vi "Day7-2.vi"() -> ()   [LabVIEW 2021]
uses:
  4c816eb8-5152-4e16-8102-76167b0c092a.vi
  <vilib>/Comparison/Less/Less Functor/Less Functor.lvclass
panel:
  out "Array 2":cluster{"path":path, i32}[](array[cluster])
  out "x-y":i32
  out "sorted array":cluster{i32, "path":path}[](array[cluster])
  out "sum 2":i32
  out "Array":cluster{"path":path, i32}[](array[cluster])
  out "array":string[][](array[string])
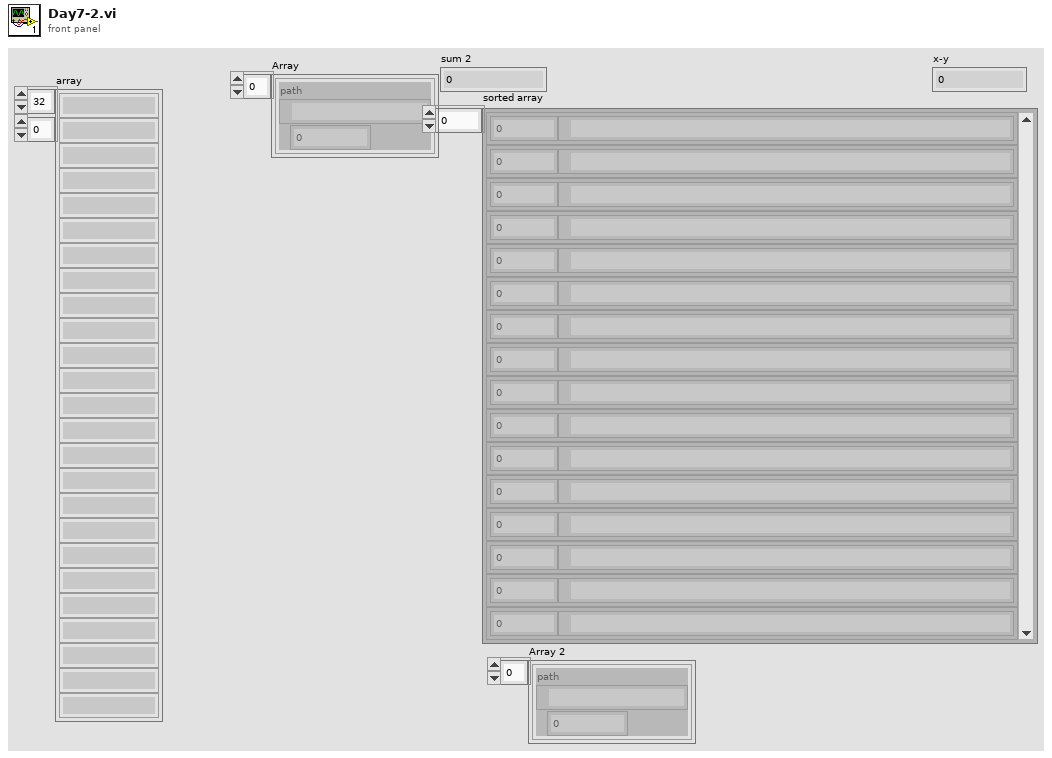
[diagram p1: front panel]
types:
  T1 = map{path, cluster{"parent directory":string, "subdirectories":string[], "contained files":cluster{"file name":string, "file size":i32}[]}}
  T2 = cluster{"parent direcotry":string, "subdirectories":string[], "contained files":cluster{"file name":string, "file size":i32}[]}
  T3 = cluster{"trimmed string":string, "file size":i32}[]
  T4 = cluster{"parent directory":string, "subdirectories":string[], "contained files":cluster{"file name":string, "file size":i32}[]}
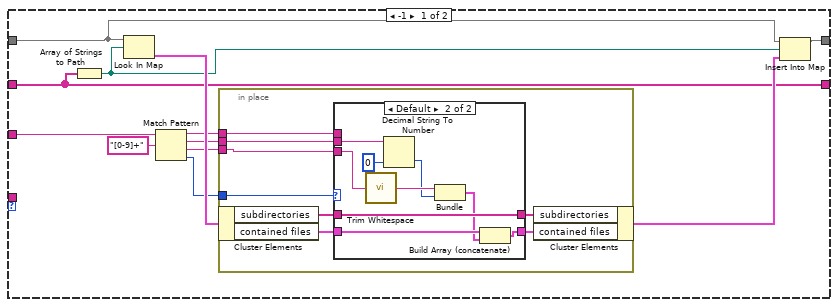
[diagram p2: hidden frame]
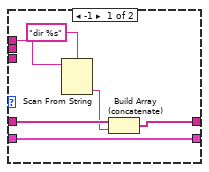
[diagram p3: hidden frame]
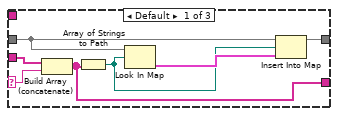
[diagram p5: hidden frame]
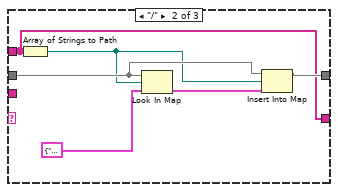
[diagram p6: hidden frame]
diagram:
  w14 = T1 {}  # Size: 0
  (unwired) "- / (dir)\n  - a (dir)\n    - e (dir)\n      - i (file, size=584)\n    - f (file, size=29116)\n    - g (file, size=2557)\n    - h.lst (file, size=62596)\n  - b.txt (file, size=14848514)\n  - c.dat (file, size=8504156)\n  - d (dir)\n    - j (file, size=4060174)\n    - d.log (file, size=8033020)\n    - d.ext (file, size=5626152)\n    - k (file, size=7214296)"
  # "directory properties\n - parent directory\n - subdirectories\n - contained files"
  # "active directory"
  n1 = Spreadsheet String To Array(format string="%s" ("spreadsheet string"), spreadsheet string="$ cd /\n$ ls\ndir ccjp\n328708 hglnvs.bsh\ndir hpsnpc\ndir pcb\ndir pntzm\ndir pzg\ndir thfgwwsp\n$ cd ccjp\n$ ls\n159990 dlz\ndir mbtsvblj\n165076 nppbjl.qhg\n$ cd mbtsvblj\n$ ls\n34806 frqsf.nsv\ndir ppq\ndir ptht\ndir rgmvdwt\n$ cd ppq\n$ ls\n266252 dhzp\n$ cd ..\n$ cd ptht\n$ ls\ndir jbnj\ndir zcbnwhzd\n$ cd jbnj\n$ ls\ndir clscr\n145780 zwtwf.zfz\n$ cd clscr\n$ ls\n249531 dhzp\n$ cd ..\n$ cd ..\n$ cd zcbnwhzd\n$ ls\ndir mbtsvblj\n$ cd mbtsvblj\n$ ls\n258527 pjhvzjt.brz\n$ cd ..\n$ cd ..\n$ cd ..\n$ cd rgmvdwt\n$ ls\n166021 hdb\n115350 ljpzpdbf\n$ cd ..\n$ cd ..\n$ cd ..\n$ cd hpsnpc\n$ ls\n6334 bfdfbrh.vff\n311949 qphlw.whm\n$ cd ..\n$ cd pcb\n$ ls\ndir ccjp\n201615 gbpzf.gmg\ndir lhth\n319302 lrmj.rmm\ndir mwl\n303062 pvftq\n$ cd ccjp\n$ ls\n10932 ccjp\n80040 jjcggmr.ljs\n299982 jrqwhsn.ptv\n280655 ljpzpdbf\n268430 mdvvj.dlf\ndir mvhhlg\ndir ppfq\ndir rdgngdm\ndir smftmb\ndir tqwchhd\n$ cd mvhhlg\n$ ls\n146902 fwhcbfr.shd\n$ cd ..\n$ cd ppfq\n$ ls\n263452 hdb\n$ cd ..\n$ cd rdgngdm\n$ ls\n46355 wlgshdgl\n$ cd ..\n$ cd smftmb\n$ ls\n56834 mhs\n325038 ppmtvcj\ndir rzcmwl\n194645 ztwqq.jfw\n$ cd rzcmwl\n$ ls\ndir btfhswwf\ndir jrd\ndir ndzfvl\n$ cd btfhswwf\n$ ls\n62811 ccjp.clj\n$ cd ..\n$ cd jrd\n$ ls\n184948 fqqg.pfc\ndir mshf\n136894 nbvbr\n$ cd mshf\n$ ls\n314602 ppmtvcj\n$ cd ..\n$ cd ..\n$ cd ndzfvl\n$ ls\n43177 hhcfpnmg.njm\n$ cd ..\n$ cd ..\n$ cd ..\n$ cd tqwchhd\n$ ls\n294014 dlz\n122061 ljpzpdbf\n54178 ppmtvcj.wlp\ndir trm\ndir zcbnwhzd\n$ cd trm\n$ ls\n279737 ccjp.mhz\n$ cd ..\n$ cd zcbnwhzd\n$ ls\n88477 dhnwjlzj\n143989 dhzp\n$ cd ..\n$ cd ..\n$ cd ..\n$ cd lhth\n$ ls\n79532 tlls\n$ cd ..\n$ cd mwl\n$ ls\ndir frc\ndir lqqqppm\n178576 prpjmrw\n$ cd frc\n$ ls\ndir cvm\n244013 dhzp\n29325 gnh\n264555 hdb\n$ cd cvm\n$ ls\n196619 hhcfpnmg.njm\n$ cd ..\n$ cd ..\n$ cd lqqqppm\n$ ls\ndir jdznl\n38505 nqv\n$ cd jdznl\n$ ls\n85492 ctt\n228912 dfbgtqj.vsb\n136077 nnwgd.vjn\n254459 zrrzsfss\n$ cd ..\n$ cd ..\n$ cd ..\n$ cd ..\n$ cd pntzm\n$ ls\ndir hnnhdd\ndir mbtsvblj\ndir vmdlwdj\n$ cd hnnhdd\n$ ls\n35908 fjp\n119221 ljpzpdbf\n210488 whhpztz.lgt\n$ cd ..\n$ cd mbtsvblj\n$ ls\ndir clfpc\ndir csqcnmtc\n18524 mbtsvblj\ndir zcrrtlh\n$ cd clfpc\n$ ls\ndir jffq\ndir qpsfrhld\n89569 tdzfqpz.wvs\n$ cd jffq\n$ ls\ndir dpngpgr\ndir htbf\n$ cd dpngpgr\n$ ls\n128899 ccjp.nbs\n$ cd ..\n$ cd htbf\n$ ls\n90381 ljpzpdbf\n$ cd ..\n$ cd ..\n$ cd qpsfrhld\n$ ls\ndir bgrb\ndir ddtlcfz\n54115 dlz\n154299 hhcfpnmg.njm\n59452 jwc.pwg\ndir mbtsvblj\n$ cd bgrb\n$ ls\n119046 ccjp.zmf\ndir qsnng\n$ cd qsnng\n$ ls\n195412 vjdh.cqv\n$ cd ..\n$ cd ..\n$ cd ddtlcfz\n$ ls\ndir ftfch\n26717 mbtsvblj\n157679 mbtsvblj.rfb\n299928 qmg\ndir trq\ndir wjhjlpr\n$ cd ftfch\n$ ls\n50242 dhzp\n58846 dlz\ndir hhwsrzhv\n$ cd hhwsrzhv\n$ ls\ndir bjnn\n67610 dhzp\ndir mbtsvblj\n205664 tmcfmshb\n$ cd bjnn\n$ ls\n199806 dlz\n$ cd ..\n$ cd mbtsvblj\n$ ls\ndir ffzjcshp\n$ cd ffzjcshp\n$ ls\ndir ppmtvcj\n$ cd ppmtvcj\n$ ls\n184744 dlz\n$ cd ..\n$ cd ..\n$ cd ..\n$ cd ..\n$ cd ..\n$ cd trq\n$ ls\n278471 ccjp\n$ cd ..\n$ cd wjhjlpr\n$ ls\ndir wzwqrfhv\n$ cd wzwqrfhv\n$ ls\n262877 ccjp\n$ cd ..\n$ cd ..\n$ cd ..\n$ cd mbtsvblj\n$ ls\n243142 ccjp.szb\n306673 lmstdpfc.nww\ndir nlsprnh\ndir nmzwtwwc\ndir rbpbl\n$ cd nlsprnh\n$ ls\n200708 stbjphg.hcs\n$ cd ..\n$ cd nmzwtwwc\n$ ls\n323366 vzq.pcj\n$ cd ..\n$ cd rbpbl\n$ ls\n59872 fmnmsjr.svf\n$ cd ..\n$ cd ..\n$ cd ..\n$ cd ..\n$ cd csqcnmtc\n$ ls\n16652 ccjp\ndir fsfd\n37144 hdb\ndir mbtsvblj\ndir mwl\n66387 nljlpbjq\ndir ppmtvcj\n120839 rgclgwnq\n$ cd fsfd\n$ ls\n105721 qqvchq.mwh\n$ cd ..\n$ cd mbtsvblj\n$ ls\ndir cdzgtll\ndir dfgd\ndir fbfr\n165975 mbtsvblj\n174541 ppmtvcj\ndir vwgrpswj\n$ cd cdzgtll\n$ ls\n163523 dhzp\n124219 dlz\n199796 hdb\n$ cd ..\n$ cd dfgd\n$ ls\n173064 ccjp.cbt\ndir cdqc\ndir fzrm\ndir grcs\n87000 mbtsvblj.zrl\ndir njvgs\ndir ppmtvcj\n210984 rhtslcwt.wgt\ndir vws\n$ cd cdqc\n$ ls\n178924 hdb\n$ cd ..\n$ cd fzrm\n$ ls\ndir bjwtbc\n211229 dhzp\ndir dtslj\n76461 mbtsvblj.mtw\n317618 mmz.mqq\ndir mwl\n163587 vwgq\n$ cd bjwtbc\n$ ls\n9891 hhcfpnmg.njm\ndir mwl\n$ cd mwl\n$ ls\n203337 glwp.dls\n112753 mwl.qph\n$ cd ..\n$ cd ..\n$ cd dtslj\n$ ls\n277817 hhcfpnmg.njm\n$ cd ..\n$ cd mwl\n$ ls\n90781 mhnrwpmg.svv\n$ cd ..\n$ cd ..\n$ cd grcs\n$ ls\n286144 rnfqhs\n$ cd ..\n$ cd njvgs\n$ ls\ndir bmhdth\ndir ccjp\ndir mwl\n$ cd bmhdth\n$ ls\n154455 ppmtvcj.hwq\n$ cd ..\n$ cd ccjp\n$ ls\n215864 fcwjtzhs.vqn\n$ cd ..\n$ cd mwl\n$ ls\n139000 fnjztz\n$ cd ..\n$ cd ..\n$ cd ppmtvcj\n$ ls\n45041 jzfnmdw.jms\ndir zstzfs\n$ cd zstzfs\n$ ls\ndir qsfsj\n$ cd qsfsj\n$ ls\n34771 rsv\n$ cd ..\n$ cd ..\n$ cd ..\n$ cd vws\n$ ls\n98036 pjs\n103603 szszjfv\n211083 ztd\n$ cd ..\n$ cd ..\n$ cd fbfr\n$ ls\ndir dshrpf\n216109 hbw.jhj\n319355 hdhl\ndir ltf\n210950 qstlgvb\ndir thhncv\n316300 zfgh\n$ cd dshrpf\n$ ls\ndir nll\ndir qrsg\n$ cd nll\n$ ls\n45935 flmvswv.rll\n4161 hhcfpnmg.njm\n82301 sww.dwj\ndir tqdmtp\n46608 tzrn.qrt\n101463 zcbnwhzd.mpm\n$ cd tqdmtp\n$ ls\n280430 dhzp\n$ cd ..\n$ cd ..\n$ cd qrsg\n$ ls\ndir htrvnvz\n$ cd htrvnvz\n$ ls\ndir mbtsvblj\n$ cd mbtsvblj\n$ ls\n235270 dlz\n$ cd ..\n$ cd ..\n$ cd ..\n$ cd ..\n$ cd ltf\n$ ls\ndir pcbc\ndir wwjnwbjj\ndir zcbnwhzd\n$ cd pcbc\n$ ls\n140010 mbtsvblj.hqd\n$ cd ..\n$ cd wwjnwbjj\n$ ls\ndir mwl\n$ cd mwl\n$ ls\ndir pddbdp\n$ cd pddbdp\n$ ls\n27497 dlz\n$ cd ..\n$ cd ..\n$ cd ..\n$ cd zcbnwhzd\n$ ls\n302364 nrgpwm.cbb\n$ cd ..\n$ cd ..\n$ cd thhncv\n$ ls\n299769 hdb\n$ cd ..\n$ cd ..\n$ cd vwgrpswj\n$ ls\ndir jgt\ndir mwl\n293673 mwl.pwl\n$ cd jgt\n$ ls\n282773 hhcfpnmg.njm\n$ cd ..\n$ cd mwl\n$ ls\n288944 jfnjdtr.ssj\n186368 wfr\ndir zrtvvf\n$ cd zrtvvf\n$ ls\n82162 gtz.gsc\n$ cd ..\n$ cd ..\n$ cd ..\n$ cd ..\n$ cd mwl\n$ ls\n98218 htc.qjr\ndir mghhqrtn\ndir qct\n$ cd mghhqrtn\n$ ls\n220446 dlz\n36230 pwwlwv.crn\n$ cd ..\n$ cd qct\n$ ls\n33534 hdb\n27140 jpwqvbs.mvr\n60637 mlqtp\n12143 nlvtp.qjn\n152733 nqjqzt\n$ cd ..\n$ cd ..\n$ cd ppmtvcj\n$ ls\ndir ccjp\n297245 zcbnwhzd\n$ cd ccjp\n$ ls\n128473 wcw.dng\n$ cd ..\n$ cd ..\n$ cd ..\n$ cd zcrrtlh\n$ ls\n27488 bcbnmhq\ndir dhsmmlt\ndir fgqbpcn\n$ cd dhsmmlt\n$ ls\n42514 cvfwqnfl\n252570 dlz\n145814 ppmtvcj.snb\n294613 rslsh.slv\n186477 vwd.spz\ndir wffbp\n$ cd wffbp\n$ ls\ndir mbtsvblj\ndir nvq\n150447 ppmtvcj.hzc\n34904 whzpsbqp.clq\ndir zcbnwhzd\n$ cd mbtsvblj\n$ ls\n65132 cmmlw.bmq\n310866 cqrtmpdp.pjq\ndir mbtsvblj\n212527 mbtsvblj.spw\n232198 ngmltt.qwl\ndir pbqh\ndir ppwgsp\ndir qqfsb\n223322 tzsmvh\n$ cd mbtsvblj\n$ ls\ndir bzpdz\ndir mbtsvblj\ndir pwnn\ndir zcbnwhzd\n$ cd bzpdz\n$ ls\n272769 gtmftv\n280597 hhcfpnmg.njm\n151008 nmgvrhr.mvp\n$ cd ..\n$ cd mbtsvblj\n$ ls\n64862 czn\n309781 dhzp\n253325 dlz\ndir dqnr\ndir fgd\n139779 ghtzv\n255567 rml.rhm\ndir srfzjfw\n$ cd dqnr\n$ ls\n302986 cjnwm.lrb\n158871 frhjlp.rnn\n180385 nrlmq\n$ cd ..\n$ cd fgd\n$ ls\n158213 msjrcl.dsh\n$ cd ..\n$ cd srfzjfw\n$ ls\ndir jfnd\n210830 ljpzpdbf\ndir mbtsvblj\ndir zcrrvpg\n$ cd jfnd\n$ ls\n300883 zvtdj.srv\n$ cd ..\n$ cd mbtsvblj\n$ ls\n287467 cjdm.whc\n233084 hpfgtnts\ndir zcbnwhzd\n$ cd zcbnwhzd\n$ ls\n79744 dlz\n$ cd ..\n$ cd ..\n$ cd zcrrvpg\n$ ls\ndir jrbcqlct\ndir srpm\n$ cd jrbcqlct\n$ ls\n325945 dlz\n$ cd ..\n$ cd srpm\n$ ls\n90698 ngw.fhm\n$ cd ..\n$ cd ..\n$ cd ..\n$ cd ..\n$ cd pwnn\n$ ls\n104826 ppmtvcj.jtm\n$ cd ..\n$ cd zcbnwhzd\n$ ls\n145508 fnr.dgt\n256683 gwdl.vfl\ndir mdv\n44255 mqdv.cdb\n79723 rgvcf\ndir sjdh\n88945 wdgq.hfm\ndir zpm\n$ cd mdv\n$ ls\n231290 dlz\n3468 hdb\n95091 mcm\n67779 mwl.ncb\ndir ppf\ndir rfwwtjdn\n143730 slrv.qdl\ndir sqbdvppf\n$ cd ppf\n$ ls\n73809 rgdtlp\n$ cd ..\n$ cd rfwwtjdn\n$ ls\n255306 dhzp\n306865 zbnmtcgr.ddf\n237019 zcbnwhzd.szn\n$ cd ..\n$ cd sqbdvppf\n$ ls\ndir ccjp\ndir mbtsvblj\n142955 str\ndir whtrbcqn\n93407 zcbnwhzd.ctr\n$ cd ccjp\n$ ls\n29914 cwtvtcnp.tft\n295537 rvlb\n$ cd ..\n$ cd mbtsvblj\n$ ls\n262652 ccjp.wbn\n297839 mbtsvblj.gnz\n249019 pqsqjg.vwr\n$ cd ..\n$ cd whtrbcqn\n$ ls\ndir ccjp\ndir hslmvvb\n51040 vzcsfcwf\n$ cd ccjp\n$ ls\n39489 slps\n$ cd ..\n$ cd hslmvvb\n$ ls\n148628 gpwnf.qtd\ndir jrl\n11814 qtjtsvgg.ltz\n$ cd jrl\n$ ls\ndir scwlmjzm\n$ cd scwlmjzm\n$ ls\n119717 vhpsrbzw.jnh\n$ cd ..\n$ cd ..\n$ cd ..\n$ cd ..\n$ cd ..\n$ cd ..\n$ cd sjdh\n$ ls\n43495 srwzspsl\n$ cd ..\n$ cd zpm\n$ ls\n137218 mwl.pzt\n$ cd ..\n$ cd ..\n$ cd ..\n$ cd pbqh\n$ ls\n202610 dlz\ndir vdrqc\n$ cd vdrqc\n$ ls\n202958 mzzmjrt\n$ cd ..\n$ cd ..\n$ cd ppwgsp\n$ ls\n248541 pzvtdl.lcc\n$ cd ..\n$ cd qqfsb\n$ ls\n211390 mbtsvblj.fvh\n241455 mwl.bzl\n$ cd ..\n$ cd ..\n$ cd nvq\n$ ls\n74730 hhcfpnmg.njm\n257109 ljpzpdbf\n8864 zcbnwhzd.ctj\n$ cd ..\n$ cd zcbnwhzd\n$ ls\n307501 ccjp\ndir dfgbztqr\ndir mwl\n248526 pmhtz\ndir rwmzdt\n$ cd dfgbztqr\n$ ls\n18261 hdb\ndir mwl\ndir ppmtvcj\n$ cd mwl\n$ ls\n36787 hdv.vfs\n283104 zrvbsht.fmm\n$ cd ..\n$ cd ppmtvcj\n$ ls\n208809 ljpzpdbf\n$ cd ..\n$ cd ..\n$ cd mwl\n$ ls\n195369 mgfvgw\n146522 mwl\n78589 sfthn\n$ cd ..\n$ cd rwmzdt\n$ ls\n10176 hdb\n$ cd ..\n$ cd ..\n$ cd ..\n$ cd ..\n$ cd fgqbpcn\n$ ls\n169227 dhzp\ndir dwsgcrz\n140391 pjjln.ngc\n162589 ppmtvcj.ngb\n199626 rcgbjn.wfv\ndir snrl\ndir vfnrs\n$ cd dwsgcrz\n$ ls\n300751 fjlw.wtp\n$ cd ..\n$ cd snrl\n$ ls\n16142 ccjp.jpw\n150389 cmbnljt.ljq\n52600 gqggd.dwm\n$ cd ..\n$ cd vfnrs\n$ ls\n217267 bwlpdfv.hzh\n$ cd ..\n$ cd ..\n$ cd ..\n$ cd ..\n$ cd vmdlwdj\n$ ls\n29199 bcgjdpj.qcj\n172894 jjgrcd.cvf\ndir ngpnmbqz\n296193 ppmtvcj.bfr\ndir tfvhhpn\n36476 wqzst.wcj\n$ cd ngpnmbqz\n$ ls\ndir gnsm\ndir ntsgrm\n$ cd gnsm\n$ ls\ndir rjzngs\ndir tvv\n$ cd rjzngs\n$ ls\ndir dpfcw\ndir spmhrb\n$ cd dpfcw\n$ ls\n181566 mgdjjd.pqg\n$ cd ..\n$ cd spmhrb\n$ ls\n163198 hhcfpnmg.njm\n$ cd ..\n$ cd ..\n$ cd tvv\n$ ls\n131443 hhcfpnmg.njm\n$ cd ..\n$ cd ..\n$ cd ntsgrm\n$ ls\n246786 dlz\n12841 pzbgrn\n$ cd ..\n$ cd ..\n$ cd tfvhhpn\n$ ls\n196923 dhzp\n$ cd ..\n$ cd ..\n$ cd ..\n$ cd pzg\n$ ls\n262706 ppbqssj.hjj\n$ cd ..\n$ cd thfgwwsp\n$ ls\ndir dsvc\ndir fbg\ndir flgmdj\n516 gwppndsl\ndir mwl\ndir qfhsr\ndir tgj\ndir wdmzc\n272804 zcbnwhzd\ndir zrfmzrl\n$ cd dsvc\n$ ls\n22089 dlz\n$ cd ..\n$ cd fbg\n$ ls\n289639 hhcfpnmg.njm\n$ cd ..\n$ cd flgmdj\n$ ls\n293793 fqrpf\n$ cd ..\n$ cd mwl\n$ ls\n159673 dhzp\ndir ftthgr\n270973 hhcfpnmg.njm\ndir jjrq\n279365 ljpzpdbf\ndir mglzfcq\n101769 pnz\n18964 rdl.wqf\n$ cd ftthgr\n$ ls\ndir ccrvnht\n170369 ljltl.slv\ndir mwl\ndir zqts\n65217 zvnhmqpz.cqb\n$ cd ccrvnht\n$ ls\n164437 hdb\n$ cd ..\n$ cd mwl\n$ ls\ndir cjsc\ndir zcbnwhzd\ndir zwzb\n$ cd cjsc\n$ ls\n91883 hhcfpnmg.njm\n203008 nfmvr\n$ cd ..\n$ cd zcbnwhzd\n$ ls\ndir mbtsvblj\n$ cd mbtsvblj\n$ ls\n187513 ljpzpdbf\n$ cd ..\n$ cd ..\n$ cd zwzb\n$ ls\n138631 ljpzpdbf\ndir sjngjp\n$ cd sjngjp\n$ ls\n52116 ccjp.ttc\n157900 fptzbpp.sdm\n89462 hhcfpnmg.njm\n$ cd ..\n$ cd ..\n$ cd ..\n$ cd zqts\n$ ls\n162402 hdb\n$ cd ..\n$ cd ..\n$ cd jjrq\n$ ls\ndir bffvw\ndir czbwf\n13447 dlz\ndir gjh\ndir hjs\n$ cd bffvw\n$ ls\n139679 dqqtq.lnb\ndir mwl\n13310 sjln.zgv\n243329 srmghrt.ffl\n72108 ssm.tph\n$ cd mwl\n$ ls\ndir fdlmfjt\ndir jms\n122108 nqwrj\n$ cd fdlmfjt\n$ ls\n75969 hdtbcsfc.vmz\n$ cd ..\n$ cd jms\n$ ls\n297556 hhcfpnmg.njm\n$ cd ..\n$ cd ..\n$ cd ..\n$ cd czbwf\n$ ls\n320541 ccjp\n$ cd ..\n$ cd gjh\n$ ls\n164281 dhzp\n286094 vjs\n$ cd ..\n$ cd hjs\n$ ls\ndir cbdzvd\n41353 ccjp\ndir gbs\n114686 hdb\ndir hmtpm\n278709 ljpzpdbf\ndir ppmtvcj\n292308 zcmlbbbc.mpp\n86096 zttwct\n$ cd cbdzvd\n$ ls\n153733 dhzp\n$ cd ..\n$ cd gbs\n$ ls\ndir nfnb\n$ cd nfnb\n$ ls\ndir hgm\n$ cd hgm\n$ ls\n233469 ljpzpdbf\n$ cd ..\n$ cd ..\n$ cd ..\n$ cd hmtpm\n$ ls\n14247 mwl\n$ cd ..\n$ cd ppmtvcj\n$ ls\ndir jcwhvcf\n241390 mwl\n$ cd jcwhvcf\n$ ls\n198254 wddq.rgp\n$ cd ..\n$ cd ..\n$ cd ..\n$ cd ..\n$ cd mglzfcq\n$ ls\ndir bsplglmj\n21700 fhflt.vgq\n56724 lpmcbzrj\n222733 qnbr\n256952 thvbqb.gtv\n$ cd bsplglmj\n$ ls\ndir zcbnwhzd\n$ cd zcbnwhzd\n$ ls\ndir mqzqz\n$ cd mqzqz\n$ ls\n75000 ppmtvcj\n$ cd ..\n$ cd ..\n$ cd ..\n$ cd ..\n$ cd ..\n$ cd qfhsr\n$ ls\n249770 gfv.cnw\n70204 qlvwhff.jhm\n$ cd ..\n$ cd tgj\n$ ls\n243926 mwl.bfv\n$ cd ..\n$ cd wdmzc\n$ ls\n19843 hdb\n264263 jbqf.str\n261303 qrvt.lbr\n$ cd ..\n$ cd zrfmzrl\n$ ls\n52067 lnfgp.nhl", array type (2D Dbl)=string[][] []) -> (array=w16:string[][])  [unwired: 1 in]
  "array" <- w16
  n2 = Index Array(array=w16, index (col)=0 ("disabled index (col)")) -> (element=w15:string[])  [unwired: 1 in]
  n3 = for {
    tunnel: w15 -> [w22] mode=indexing
    shift-right: [w23] -> _
    shift-left: string[] [] ("array of strings") -> [w24]
    shift-right: [w20] -> w13
    shift-left: w14 -> [w21]
    n4 = Match Pattern(string=w22, regular expression="^\\$") -> (after substring=w25:string, offset past match=w26:i32)  [unwired: 1 in, 2 out]
    n5 = case shown="Default" w26 {
      tunnel: w22 -> [w39 w69]
      tunnel: w25 -> [_ w73]
      tunnel: w24 -> [w29 w68]
      tunnel: [w29 w66] -> w23
      tunnel: w21 -> [w36 w65]
      tunnel: [w35 w64] -> w20
      frame -1 {
        n6 = Array of Strings to Path(0:w29) -> (2:w28:path)  [unwired: 1 in]
        n7 = Look In Map(map=w36, key=w28) -> (value=w37:T2)  [unwired: 1 in, 1 out]
        n8 = Match Pattern(string=w39, regular expression="[0-9]+") -> (before substring=w32:string, match substring=w31:string, after substring=w30:string, offset past match=w33:i32)  [unwired: 1 in]
        n9 = in-place {
          in-place-border: w33 -> [w47]
          in-place-border: w32 -> [w46]
          in-place-border: w31 -> [w41]
          in-place-border: w30 -> [w40]
          n10 = in-place-cluster #1(w37) -> ("subdirectories"=w45:string[], "contained files"=w42:cluster{"file name":string, "file size":i32}[])
          n11 = case shown="Default" w47 {
            tunnel: w46 -> [w53 _]
            tunnel: w45 -> [w51 w62]
            tunnel: [w49 w62] -> w44
            tunnel: [w48 w54] -> w43
            tunnel: w42 -> [w48 w56]
            tunnel: w41 -> [_ w61]
            tunnel: w40 -> [_ w60]
            frame -1 {
              n12 = Scan From String(format string="dir %s", input string=w53) -> (output 1=w50:string)  [unwired: 3 in, 3 out]
              n13 = Build Array (concatenate)(w51, w50) -> (w49:string[])
            }
            frame Default {
              n14 = call <vilib>:"Trim Whitespace.vi"("string"=w60) -> ("trimmed string"=w58:string)  [unwired: 1 in]
              n15 = Decimal String To Number(string=w61, default (0L)=0 ("default (0 I32)")) -> (number=w57:i32)  [unwired: 1 in, 1 out]
              n16 = Bundle("trimmed string"=w58, w57) -> (w55:cluster{"trimmed string":string, i32})  [unwired: 1 in]
              n17 = Build Array (concatenate)(w56, w55) -> (w54:T3)
            }
          }
          n18 = in-place-cluster #1("subdirectories"=w44, "contained files"=w43) -> (w34:T2)
        }
        n19 = Insert Into Map(map in=w36, key=w28, value=w34) -> (map out=w35:T1)  [unwired: 2 out]
      }
      frame Default {
        # "This is a command"
        n20 = call <vilib>:"Trim Whitespace.vi"("string"=w73) -> ("trimmed string"=w72:string)  [unwired: 1 in]
        n21 = call <vilib>:"Space Constant.vi"() -> ("String"=w71:string)
        n22 = Search/Split String(string=w72, search string/char (-)=w71) -> (substring before match=w70:string, match + rest of string=w67:string)  [unwired: 1 in, 1 out]
        n23 = case shown="\"cd\"" w70 {
          tunnel: w69 -> [_ _ _]
          tunnel: w68 -> [w75 w79 w100]
          tunnel: w67 -> [_ w82 _]
          tunnel: [w75 w80 w100] -> w66
          tunnel: w65 -> [w74 w78 w99]
          tunnel: [w74 w77 w99] -> w64
          tunnel: string[] ["root"] ("array of strings") -> [_ w76 _]
          frame Default {
          }
          frame "cd" {
            n24 = call <vilib>:"Trim Whitespace.vi"("string"=w82) -> ("trimmed string"=w81:string)  [unwired: 1 in]
            n25 = case shown="\"..\"" w81 {
              selector: w81 -> [w87 _ _]
              tunnel: [w83 w90 w96] -> w80
              tunnel: w79 -> [w86 _ w97]
              tunnel: w78 -> [w88 w94 w98]
              tunnel: [w89 w93 w98] -> w77
              tunnel: w76 -> [_ w90 _]
              frame Default {
                n26 = Build Array (concatenate)(w86, w87) -> (w83:string[])
                n27 = Array of Strings to Path(0:w83) -> (2:w84:path)  [unwired: 1 in]
                n28 = Look In Map(map=w88, key=w84) -> (value=w85:T4)  [unwired: 1 in, 1 out]
                n29 = Insert Into Map(map in=w88, key=w84, value=w85) -> (map out=w89:T1)  [unwired: 2 out]
              }
              frame "/" {
                n30 = Array of Strings to Path(0:w90) -> (2:w91:path)  [unwired: 1 in]
                n31 = Look In Map(map=w94, key=w91, default value=T2 {"parent direcotry"="", "subdirectories"=[], "contained files"=[]}) -> (value=w92:T2)  [unwired: 1 out]
                n32 = Insert Into Map(map in=w94, key=w91, value=w92) -> (map out=w93:T1)  [unwired: 2 out]
              }
              frame ".." {
                n33 = Delete From Array(array=w97) -> (array with subset deleted=w96:string[])  [unwired: 2 in, 1 out]
              }
            }
          }
          frame "ls" {
          }
        }
      }
    }
  }
  n34 = for {
    tunnel: w13 -> [w113] mode=indexing
    tunnel: w13 -> [w111]
    tunnel: [w102] -> w10 mode=indexing
    tunnel: [w101] -> w11 mode=indexing
    n35 = Unbundle By Name(w113) -> ("path"=w104:path)
    n36 = Look In Map(map=w111, key=w104) -> (value=w112:T4)  [unwired: 1 in, 1 out]
    n37 = Unbundle By Name(w112) -> ("subdirectories"=w105:string[], "contained files"=w110:cluster{"file name":string, "file size":i32}[])
    n38 = for {
      tunnel: w105 -> [w116] mode=indexing
      tunnel: w104 -> [w115]
      tunnel: [w114] -> w103 mode=indexing
      n39 = Build Path(base path=w115, name or relative path=w116) -> (appended path=w114:path)
    }
    n40 = while {
      tunnel: w111 -> [w131]
      shift-right: [w124] -> _
      shift-left: w103 -> [w127]
      tunnel: [w122] -> w108 mode=indexing
      stop <- w123 stop-if-true
      n41 = Delete From Array(array=w127, index=0) -> (deleted portion=w120:path, array with subset deleted=w125:path[])  [unwired: 1 in]
      n42 = Look In Map(map=w131, key=w120) -> (value=w130:T4)  [unwired: 1 in, 1 out]
      n43 = Unbundle By Name(w130) -> ("subdirectories"=w121:string[], "contained files"=w128:cluster{"file name":string, "file size":i32}[])
      n44 = for {
        tunnel: w121 -> [w134] mode=indexing
        tunnel: w120 -> [w133]
        tunnel: [w132] -> w119 mode=indexing
        n45 = Build Path(base path=w133, name or relative path=w134) -> (appended path=w132:path)
      }
      n46 = Build Array (concatenate)(w125, w119) -> (w124:path[])
      n47 = for {
        tunnel: w128 -> [w136] mode=indexing
        tunnel: [w135] -> w129 mode=indexing
        n48 = Unbundle By Name(w136) -> ("file size"=w135:i32)
      }
      n49 = Empty Array?(array=w124) -> (empty?=w123:bool)
      n50 = Add Array Elements(numeric array=w129) -> (sum=w122:i32)
    }
    n51 = for {
      tunnel: w110 -> [w118] mode=indexing
      tunnel: [w117] -> w109 mode=indexing
      n52 = Unbundle By Name(w118) -> ("file size"=w117:i32)
    }
    n53 = Add Array Elements(numeric array=w109) -> (sum=w101:i32)
    n54 = Add Array Elements(numeric array=w108) -> (sum=w107:i32)
    n55 = Add(x=w107, y=w101) -> (x+y=w106:i32)
    n56 = Bundle("path"=w104, w106) -> (w102:cluster{"path":path, i32})  [unwired: 1 in]
  }
  "Array" <- w10
  n57 = Add Array Elements(numeric array=w11) -> (sum=w6:i32)
  "sum 2" <- w6
  n58 = for {
    tunnel: w10 -> [w140] mode=indexing
    tunnel: [w137] -> w9 mode=indexing
    n59 = Unbundle(w140) -> ("path"=w138:path, w139:i32)
    n60 = Bundle(w139, "path"=w138) -> (w137:cluster{i32, "path":path})  [unwired: 1 in]
  }
  n61 = Subtract(x=70000000, y=w6) -> (x-y=w3:i32)
  n62 = Subtract(x=30000000, y=w3) -> (x-y=→"x-y":i32)
  n63 = call "Sort 1D Array.vim"("unsorted array"=w9) -> ("sorted array"=w8:cluster{i32, "path":path}[])  [unwired: 10 in]
  n64 = Reverse 1D Array(array=w8) -> (reversed array=→"sorted array":cluster{i32, "path":path}[])
